vi "Configure RX Port FIFO.vi"(0 "Refnum in":refnum<k20>, 5 "RX Port":T1 items=["Port 0", "Port 1", "Port 2", "Port 3"], 7 "FIFO Depth":u32, 11 "error in":errorcluster) -> (4 "Refnum out":refnum<k20>, 6 "Actual Depth":u32, 15 "error out":errorcluster)   [LabVIEW 2016, in "Aurora Stream (NI 6592R) (Host).lvlib"]
doc: "Configures the FIFO connected to the specified port and starts the FIFO.\n\n<B>Input Parameters</B>\n\n<B>Refnum in</B> Receives a reference to the FPGA from the previous VI.\n\n<B>RX Port</B> Identifies the physical port whose project resources will be configured.\n\n<B>FIFO Depth</B> Specifies the number of elements to allocate for the host-side FIFO buffer.\n\n<B>error in</B> describes error conditions that occur before this node runs. This input provides standard error in functionality.\n\n<B>Output Parameters</B>\n\n<B>Refnum out</B> passes a reference to the FPGA to the next VI.\n\n<B>error out</B> contains error information. This output provides standard error out functionality."
uses:
  Aurora Stream (NI 6592R) (Host).lvlib
  Port.ctl
  Base Bitfile Reference.ctl
  <vilib>/rvi/interface/common/niFpgaWaitOnOcc.vi
  <vilib>/Utility/error.llb/Error Cluster From Error Code.vi
  <vilib>/rvi/interface/nirviMethod/nirviMethod.xnode
  <vilib>/FPGAPlugInAG/Dynamic/niLvFpga_ConfigureFifo_Dynamic.vi
  <vilib>/rvi/errors/niLvFpgaMergeErrorWithErrorCode.vi
  <vilib>/FPGAPlugInAG/Dynamic/niLvFpga_StartFifo_Dynamic.vi
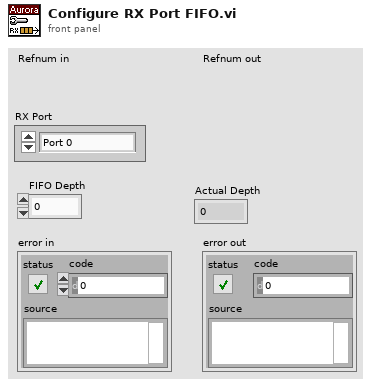
[diagram p1: front panel]
types:
  T1 = typedef "Aurora Stream (NI 6592R) (Host).lvlib/Port.ctl" = i32
  T2 = typedef "Aurora Stream (NI 6592R) (Host).lvlib/Base Bitfile Reference.ctl" = refnum<k20>
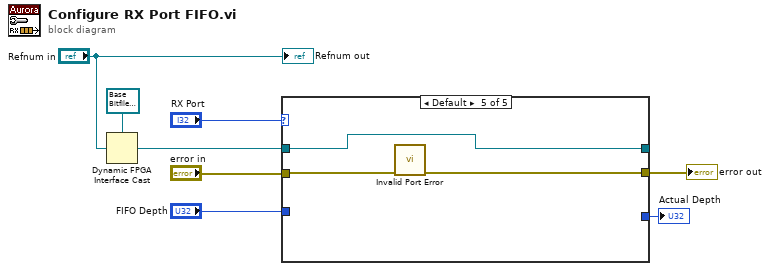
[diagram p0: block diagram]
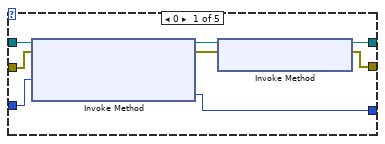
[diagram p2: hidden frame]
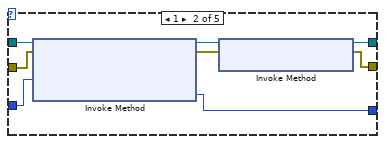
[diagram p3: hidden frame]
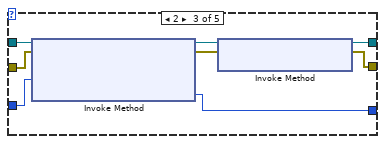
[diagram p4: hidden frame]
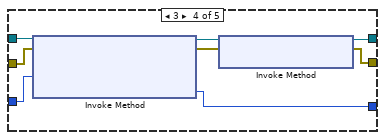
[diagram p5: hidden frame]
diagram:
  n1 = Dynamic FPGA Interface Cast(Session In=T2 refnum ("Aurora Sample Project"), Type="Refnum in") -> (Session Out=w3:T2)
  n2 = case shown="Default" "RX Port" {
    tunnel: [w10 w19 w26 w34 w41] -> w6
    tunnel: w3 -> [w16 w22 w32 w38 w43]
    tunnel: "error in" -> [w15 w21 w31 w36 w42]
    tunnel: [w11 w20 w28 w35 w43] -> _
    tunnel: "FIFO Depth" -> [w14 w18 w30 w37 _]
    tunnel: [w9 w17 w25 w33 _] -> w1
    frame 0 {
      n3 = xnode "Invoke Method"("FPGA VI Reference In"=w16, "error in"=w15, "Requested Depth"=w14) -> ("FPGA VI Reference Out"=w13:T2, "error out"=w12:errorcluster, "Actual Depth"=w9:u32)
      n4 = xnode "Invoke Method"("FPGA VI Reference In"=w13, "error in"=w12) -> ("FPGA VI Reference Out"=w11:T2, "error out"=w10:errorcluster)
    }
    frame 1 {
      n5 = xnode "Invoke Method"("FPGA VI Reference In"=w22, "error in"=w21, "Requested Depth"=w18) -> ("FPGA VI Reference Out"=w24:T2, "error out"=w23:errorcluster, "Actual Depth"=w17:u32)
      n6 = xnode "Invoke Method"("FPGA VI Reference In"=w24, "error in"=w23) -> ("FPGA VI Reference Out"=w20:T2, "error out"=w19:errorcluster)
    }
    frame 2 {
      n7 = xnode "Invoke Method"("FPGA VI Reference In"=w32, "error in"=w31, "Requested Depth"=w30) -> ("FPGA VI Reference Out"=w29:T2, "error out"=w27:errorcluster, "Actual Depth"=w25:u32)
      n8 = xnode "Invoke Method"("FPGA VI Reference In"=w29, "error in"=w27) -> ("FPGA VI Reference Out"=w28:T2, "error out"=w26:errorcluster)
    }
    frame 3 {
      n9 = xnode "Invoke Method"("FPGA VI Reference In"=w38, "error in"=w36, "Requested Depth"=w37) -> ("FPGA VI Reference Out"=w40:T2, "error out"=w39:errorcluster, "Actual Depth"=w33:u32)
      n10 = xnode "Invoke Method"("FPGA VI Reference In"=w40, "error in"=w39) -> ("FPGA VI Reference Out"=w35:T2, "error out"=w34:errorcluster)
    }
    frame Default {
      n11 = call "Invalid Port Error.vi"("error in"=w42) -> ("error out"=w41:errorcluster)  [unwired: 14 in]
    }
  }
  "error out" <- w6
  "Actual Depth" <- w1
  "Refnum out" <- "Refnum in"
